vi "get_control.vi"(11 "path":string) -> (0 "error out":errorcluster, 3 "enum_frontpanel_image":picture)   [LabVIEW 2026]
doc: "Returns a screenshot of the content (frontpanel) of a .ctl file. Use this to understand the content of a LabVIEW type definition or custom control."
uses:
  G-AI Core/G-AI Core.lvlib
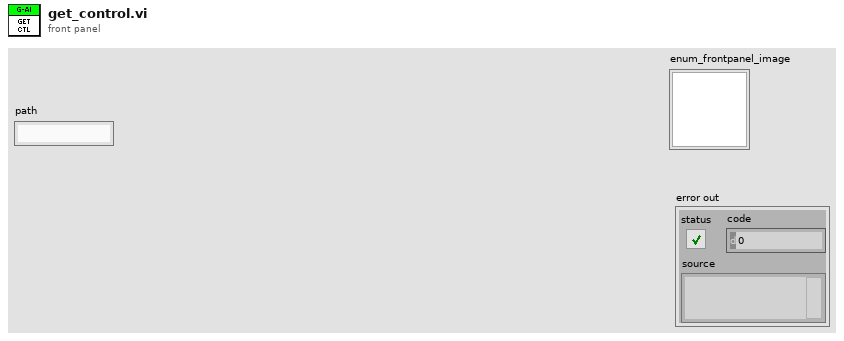
[diagram p1: front panel]
types:
  T1 = typedef "imagedata.ctl" = cluster{"image type":i32, "image depth":i32, "image":u8[], "mask":u8[], "colors":u32[], "Rectangle":cluster{"left":i16, "top":i16, "right":i16, "bottom":i16}}
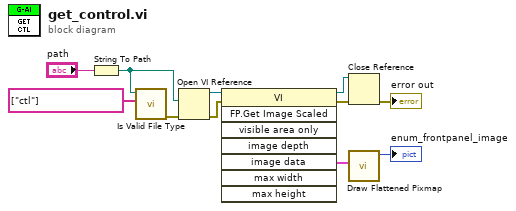
[diagram p0: block diagram]
diagram:
  n1 = String To Path(string="path") -> (path=w3:path)
  n2 = call "Is Valid File Type.vi"("y"=string[] ["ctl"], "Path"=w3) -> ("error out"=w1:errorcluster)  [unwired: 9 in]
  n3 = Open VI Reference(vi path=w3, error in (no error)=w1) -> (vi reference=w9:refnum<vi>, error out=w8:errorcluster)  [unwired: 4 in]
  n4 = invoke class="VI" method="FP.Get Image Scaled"(reference=w9, error in=w8) -> (reference out=w6:refnum<vi>, error out=w7:errorcluster, "image data"=w10:T1)  [unwired: 6 in, 5 out]
  n5 = Close Reference(reference=w6, error in (no error)=w7) -> (error out=→"error out":errorcluster)
  n6 = call <vilib>:"Draw Flattened Pixmap.vi"("image data"=w10) -> ("new picture"=→"enum_frontpanel_image":picture)  [unwired: 8 in]
